vi "Calculator-teardown.vi"(7 "test case ID":string, 8 "error in (no error)":errorcluster, 11 "result":dbl) -> (3 "result":bool)   [LabVIEW 2015]
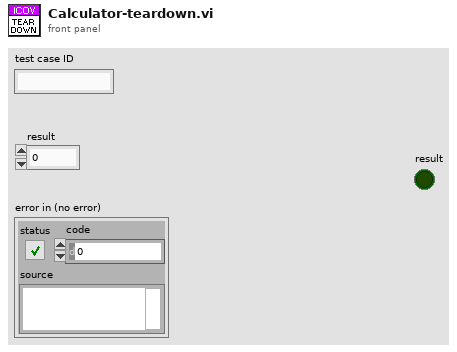
[diagram p1: front panel]
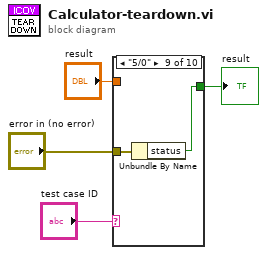
[diagram p0: block diagram]
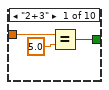
[diagram p2: hidden frame]
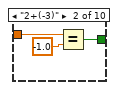
[diagram p3: hidden frame]
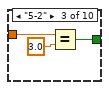
[diagram p4: hidden frame]
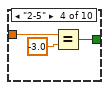
[diagram p5: hidden frame]
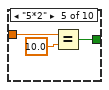
[diagram p6: hidden frame]
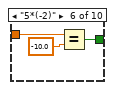
[diagram p7: hidden frame]
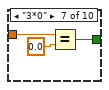
[diagram p8: hidden frame]
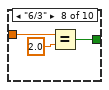
[diagram p9: hidden frame]
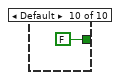
[diagram p10: hidden frame]
diagram:
  n1 = case shown="\"5/0\"" "test case ID" {
    tunnel: "error in (no error)" -> [_ _ _ _ _ _ _ _ w30 _]
    tunnel: "result" -> [w6 w10 w13 w15 w19 w22 w25 w28 _ _]
    tunnel: [w5 w8 w11 w14 w17 w21 w23 w26 w29 FALSE] -> w1
    frame "2+3" {
      n2 = Equal?(x=w6, y=5.0) -> (x = y?=w5:bool)
    }
    frame "2+(-3)" {
      n3 = Equal?(x=w10, y=-1.0) -> (x = y?=w8:bool)
    }
    frame "5-2" {
      n4 = Equal?(x=w13, y=3.0) -> (x = y?=w11:bool)
    }
    frame "2-5" {
      n5 = Equal?(x=w15, y=-3.0) -> (x = y?=w14:bool)
    }
    frame "5*2" {
      n6 = Equal?(x=w19, y=10.0) -> (x = y?=w17:bool)
    }
    frame "5*(-2)" {
      n7 = Equal?(x=w22, y=-10.0) -> (x = y?=w21:bool)
    }
    frame "3*0" {
      n8 = Equal?(x=w25, y=0.0) -> (x = y?=w23:bool)
    }
    frame "6/3" {
      n9 = Equal?(x=w28, y=2.0) -> (x = y?=w26:bool)
    }
    frame "5/0" {
      n10 = Unbundle By Name(w30) -> ("status"=w29:bool)
    }
    frame Default {
    }
  }
  "result" <- w1
